vi "DeviceConfigurationUpdateRoutedMessage_Parse.vi"(8 "error in (no error)":errorcluster, 11 "Message":T18) -> (0 "error out":errorcluster, 1 "Body":T1, 2 "Header":T17, 3 "DeviceConfigurationUpdateRoutedMessage":T16)   [LabVIEW 2017]
uses:
  <vilib>/addons/InsightCM/MessageBus/Base/controls/Message.ctl
  <vilib>/addons/InsightCM/MessageBus/Base/controls/MessageHeader.ctl
  <vilib>/addons/InsightCM/MessageBus/Base/controls/KeyValuePair.ctl
  <vilib>/addons/InsightCM/MessageBus/MessageLibrary/Device/controls/DeviceConfigurationUpdateRoutedMessage.ctl
  <vilib>/addons/InsightCM/MessageBus/MessageLibrary/Device/controls/DeviceConfigurationUpdateRoutedMessageBody.ctl
  <vilib>/addons/InsightCM/MessageBus/Base/controls/DeviceProvisioning.ctl
  <vilib>/addons/InsightCM/MessageBus/Base/controls/DeviceModel.ctl
  <vilib>/addons/InsightCM/MessageBus/Base/controls/Device.ctl
  <vilib>/addons/InsightCM/MessageBus/Base/controls/DeviceState.ctl
  <vilib>/addons/InsightCM/MessageBus/Base/controls/DataGroup.ctl
  <vilib>/addons/InsightCM/MessageBus/Base/controls/BurstModeTrigger.ctl
  <vilib>/addons/InsightCM/MessageBus/Base/controls/Trigger.ctl
  <vilib>/addons/InsightCM/MessageBus/Base/controls/Condition.ctl
  <vilib>/addons/InsightCM/MessageBus/Base/controls/DeviceSensorGroup.ctl
  <vilib>/addons/InsightCM/MessageBus/Base/controls/WirelessEndpoint.ctl
  <vilib>/addons/InsightCM/MessageBus/Base/controls/WirelessChannel.ctl
  <vilib>/addons/InsightCM/MessageBus/Base/controls/Channel.ctl
  <vilib>/addons/InsightCM/MessageBus/Base/controls/Tag.ctl
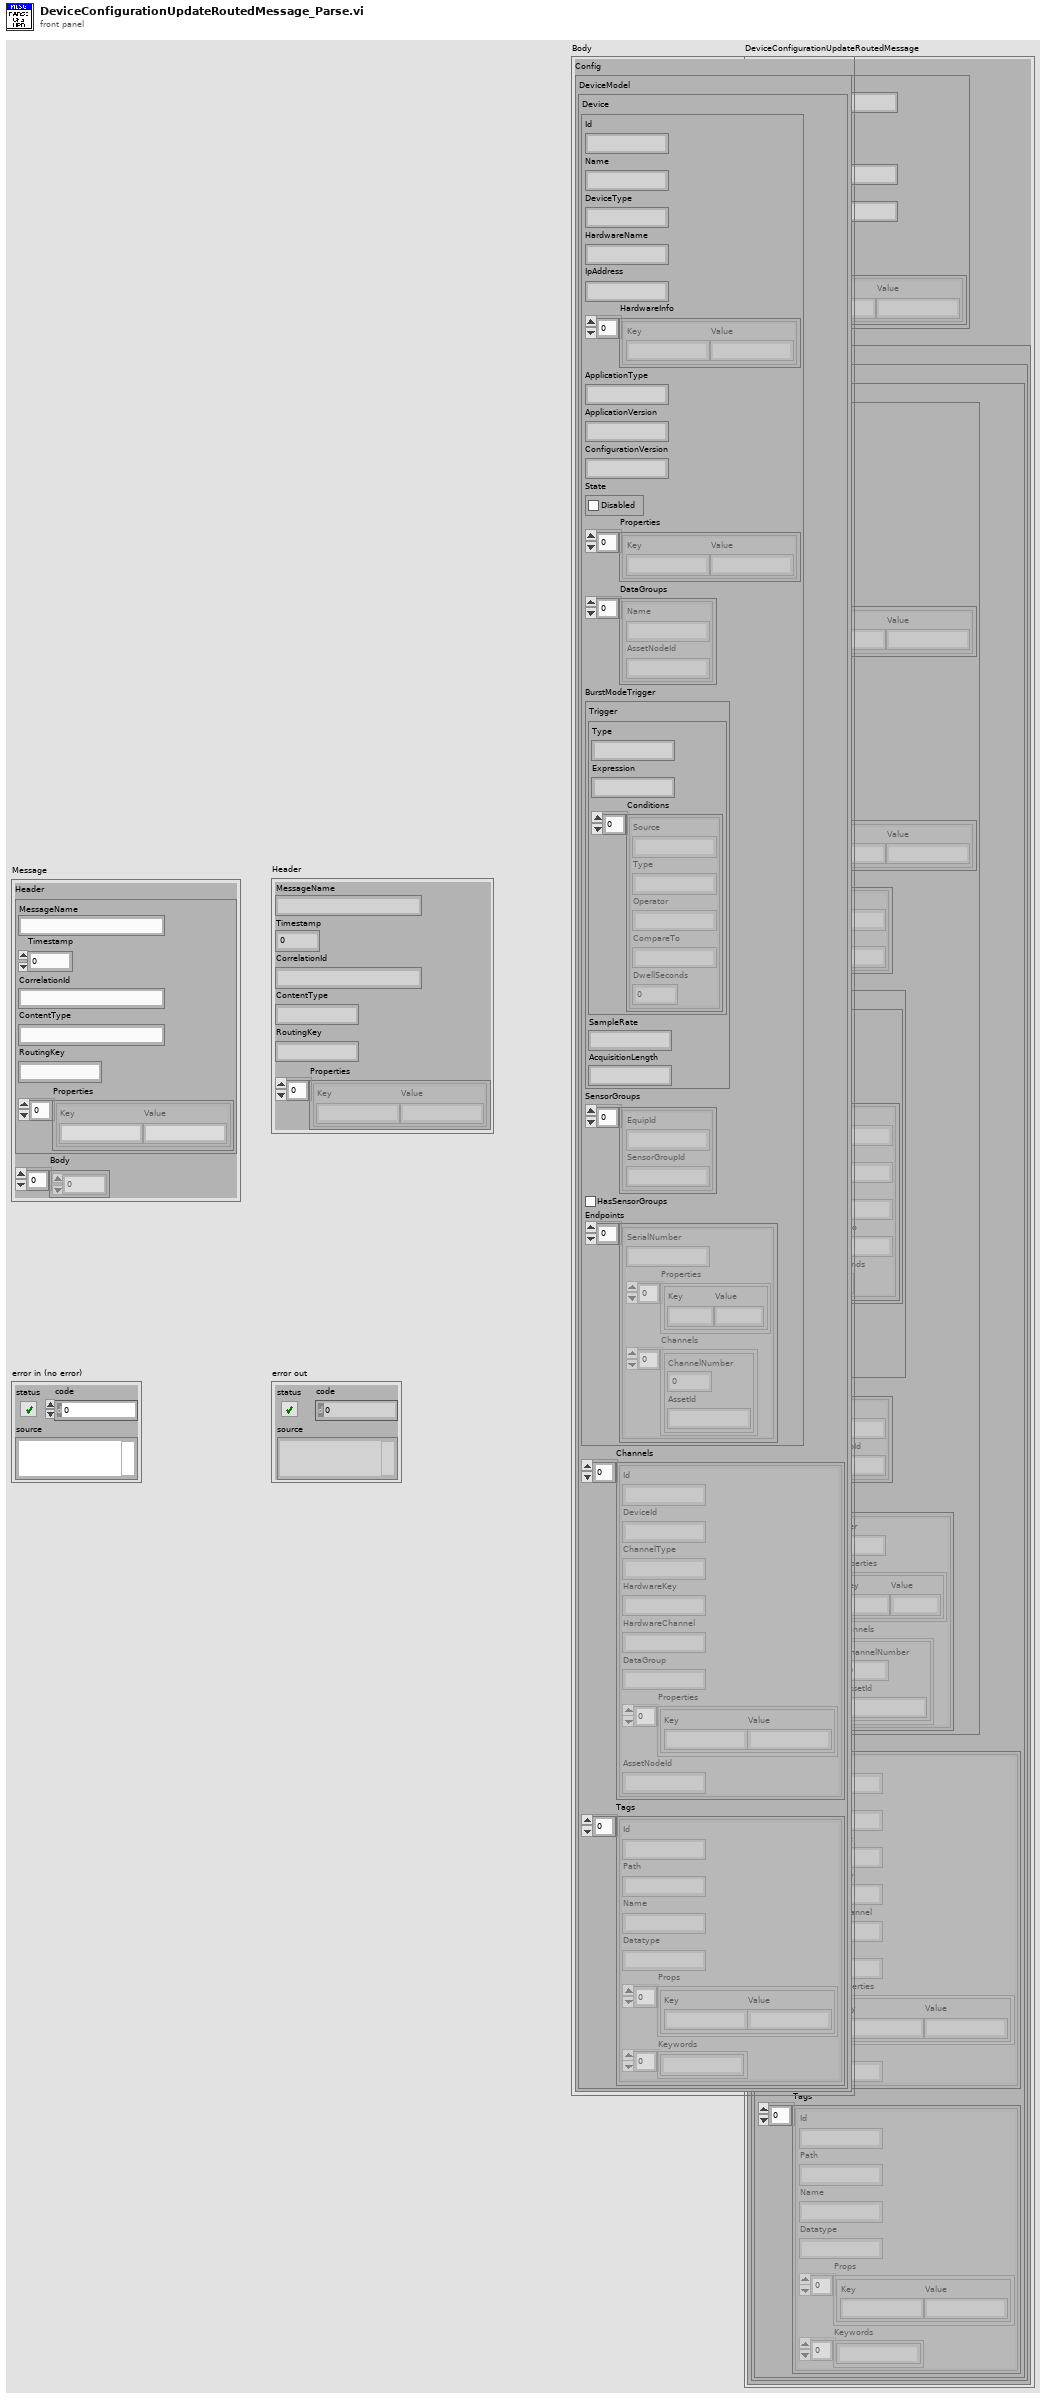
[diagram p1: front panel]
types:
  T1 = typedef "DeviceConfigurationUpdateRoutedMessageBody.ctl" = cluster{"Config":T2}
  T2 = typedef "DeviceProvisioning.ctl" = cluster{"DeviceModel":T3}
  T3 = typedef "DeviceModel.ctl" = cluster{"Device":T4, "Channels":T14[], "Tags":T15[]}
  T4 = typedef "Device.ctl" = cluster{"Id":string, "Name":string, "DeviceType":string, "HardwareName":string, "IpAddress":string, "HardwareInfo":T5[], "ApplicationType":string, "ApplicationVersion":string, "ConfigurationVersion":string, "State":T6, "Properties":T5[], "DataGroups":T7[], "BurstModeTrigger":T8, "SensorGroups":T11[], "HasSensorGroups":bool, "Endpoints":T12[]}
  T5 = typedef "KeyValuePair.ctl" = cluster{"Key":string, "Value":string}
  T6 = typedef "DeviceState.ctl" = cluster{"Disabled":bool}
  T7 = typedef "DataGroup.ctl" = cluster{"Name":string, "AssetNodeId":string}
  T8 = typedef "BurstModeTrigger.ctl" = cluster{"Trigger":T9, "SampleRate":string, "AcquisitionLength":string}
  T9 = typedef "Trigger.ctl" = cluster{"Type":string, "Expression":string, "Conditions":T10[]}
  T10 = typedef "Condition.ctl" = cluster{"Source":string, "Type":string, "Operator":string, "CompareTo":string, "DwellSeconds":dbl}
  T11 = typedef "DeviceSensorGroup.ctl" = cluster{"EquipId":string, "SensorGroupId":string}
  T12 = typedef "WirelessEndpoint.ctl" = cluster{"SerialNumber":string, "Properties":T5[], "Channels":T13[]}
  T13 = typedef "WirelessChannel.ctl" = cluster{"ChannelNumber":i32, "AssetId":string}
  T14 = typedef "Channel.ctl" = cluster{"Id":string, "DeviceId":string, "ChannelType":string, "HardwareKey":string, "HardwareChannel":string, "DataGroup":string, "Properties":T5[], "AssetNodeId":string}
  T15 = typedef "Tag.ctl" = cluster{"Id":string, "Path":string, "Name":string, "Datatype":string, "Props":T5[], "Keywords":string[]}
  T16 = typedef "DeviceConfigurationUpdateRoutedMessage.ctl" = cluster{"Header":T17, "Body":T1}
  T17 = typedef "MessageHeader.ctl" = cluster{"MessageName":string, "Timestamp":i64, "CorrelationId":string, "ContentType":string, "RoutingKey":string, "Properties":T5[]}
  T18 = typedef "Message.ctl" = cluster{"Header":T17, "Body":u8[]}
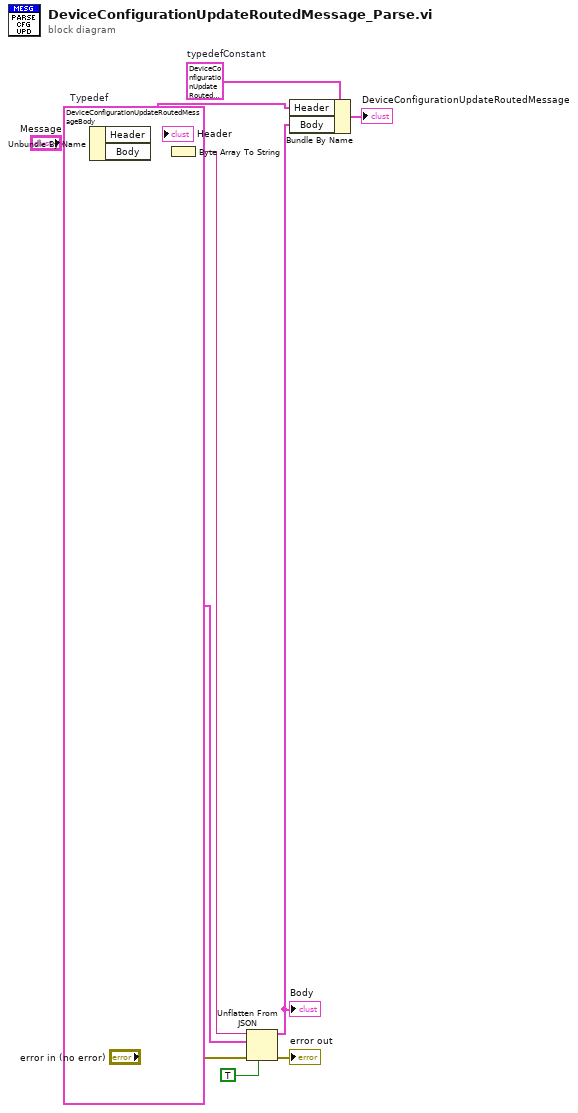
[diagram p0: block diagram]
diagram:
  w3 = T16 {"Header"={"MessageName"="", "Timestamp"=0, "CorrelationId"="", "ContentType"="", "RoutingKey"="", "Properties"=[]}, "Body"={"Config"={"DeviceModel"={"Device"={"Id"="", "Name"="", "DeviceType"="", "HardwareName"="", "IpAddress"="", "HardwareInfo"=[], "ApplicationType"="", "ApplicationVersion"="", "ConfigurationVersion"="", "State"={"Disabled"=FALSE}, "Properties"=[], "DataGroups"=[], "BurstModeTrigger"={"Trigger"={"Type"="", "Expression"="", "Conditions"=[]}, "SampleRate"="", "AcquisitionLength"=""}, "SensorGroups"=[], "HasSensorGroups"=FALSE, "Endpoints"=[]}, "Channels"=[], "Tags"=[]}}}}  # typedefConstant
  w7 = T1 {"Config"={"DeviceModel"={"Device"={"Id"="", "Name"="", "DeviceType"="", "HardwareName"="", "IpAddress"="", "HardwareInfo"=[], "ApplicationType"="", "ApplicationVersion"="", "ConfigurationVersion"="", "State"={"Disabled"=FALSE}, "Properties"=[], "DataGroups"=[], "BurstModeTrigger"={"Trigger"={"Type"="", "Expression"="", "Conditions"=[]}, "SampleRate"="", "AcquisitionLength"=""}, "SensorGroups"=[], "HasSensorGroups"=FALSE, "Endpoints"=[]}, "Channels"=[], "Tags"=[]}}}  # Typedef
  n1 = Unbundle By Name("Message") -> ("Header"=w9:T17, "Body"=w1:u8[])
  "Header" <- w9
  n2 = Byte Array To String(unsigned byte array=w1) -> (string=w6:string)
  n3 = Unflatten From JSON(JSON string=w6, type and defaults=w7, default null elements? (F)=TRUE, error in (no error)="error in (no error)") -> (value=w5:T1, error out=→"error out":errorcluster)  [unwired: 3 in]
  "Body" <- w5
  n4 = Bundle By Name(cluster=w3, "Header"=w9, "Body"=w5) -> (→"DeviceConfigurationUpdateRoutedMessage":T16)
